vi "Disk On.vi"(0 "Notifier Name":string, 11 "Error In":errorcluster) -> (4 "Notifier Name Dup":string, 8 "Disk On?":bool, 15 "Error Out":errorcluster)   [LabVIEW 2020]
uses:
  Spinning Disk Type Defs/SD Notifer Data.ctl
  Spinning Disk Type Defs/SD Actions.ctl
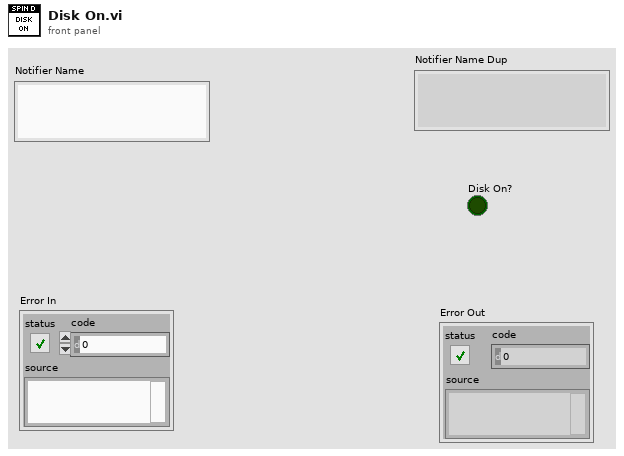
[diagram p1: front panel]
types:
  T1 = typedef "SD Notifer Data.ctl" = cluster{"Actions":T2, "Disk On?":bool, "Dichroic Pos.":i32, "Filter Wheel Pos.":i32, "Disk Pos.":i32, "Recived":bool, "Num Pos":i32[]}
  T2 = typedef "SD Actions.ctl" = enum16{"Status", "Get All Pos.", "Get Num. Pos.", "Home All", "Set Filter Wheel Pos.", "Set Disk Pos.", "Set Dichroic Pos.", "Disk On", "Disk Off", "Quit"}
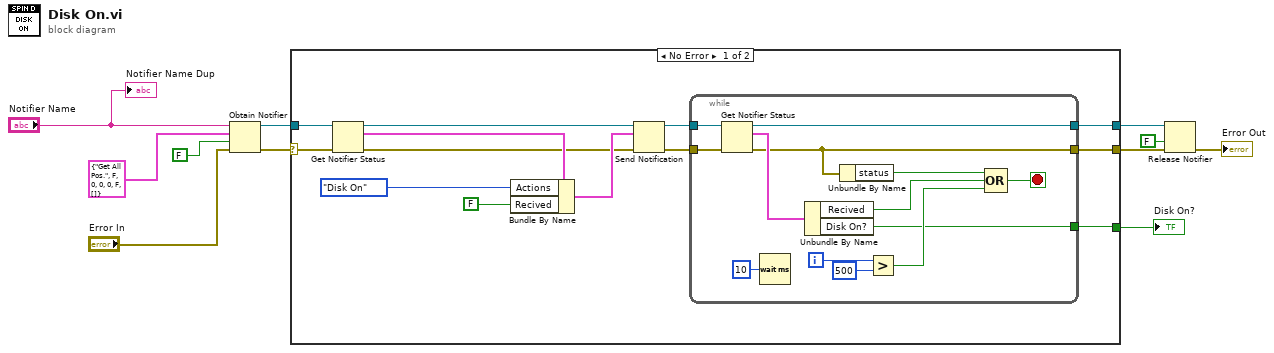
[diagram p0: block diagram]
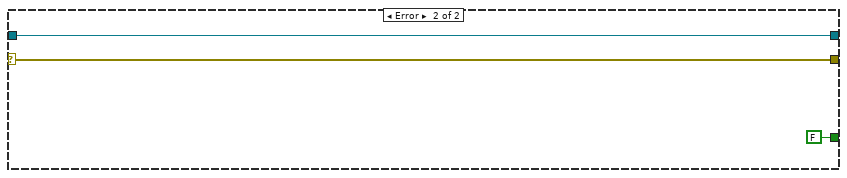
[diagram p2: hidden frame]
diagram:
  n1 = Obtain Notifier(name (unnamed)="Notifier Name", notification data type=T1 {"Actions"=enum."Get All Pos.", "Disk On?"=FALSE, "Dichroic Pos."=0, "Filter Wheel Pos."=0, "Disk Pos."=0, "Recived"=FALSE, "Num Pos"=[]} ("XLight Notifier Data"), create if not found? (T)=FALSE, error in (no error)="Error In") -> (notifier out=w7:refnum<notifier>, error out=w4:errorcluster)  [unwired: 1 out]
  n2 = case shown="No Error" w4 {
    selector: w4 -> [w23 w39]
    tunnel: w7 -> [w24 w40]
    tunnel: [w13 w40] -> w6
    tunnel: [w14 w39] -> w3
    tunnel: [w12 FALSE ("Disk On?")] -> w1
    frame No Error {
      n3 = Get Notifier Status(notifier=w24, error in (no error)=w23) -> (notifier out=w19:refnum<notifier>, current notification=w22:T1, error out=w17:errorcluster)  [unwired: 2 out]
      n4 = Bundle By Name(cluster=w22, "Actions"=SD_Actions."Disk On", "Recived"=FALSE) -> (w18:T1)
      n5 = Send Notification(notification=w18, notifier=w19, error in (no error)=w17) -> (notifier out=w16:refnum<notifier>, error out=w15:errorcluster)
      n6 = while {
        tunnel: w16 -> [w35]
        tunnel: w15 -> [w34]
        tunnel: [w28] -> w14
        tunnel: [w27] -> w13
        tunnel: [w26] -> w12
        i -> [w37]
        stop <- w29 stop-if-true
        n7 = Get Notifier Status(notifier=w35, error in (no error)=w34) -> (notifier out=w27:refnum<notifier>, current notification=w33:T1, error out=w28:errorcluster)  [unwired: 2 out]
        n8 = Wait (ms)(milliseconds to wait=u32 10) -> ()  [unwired: 1 out]
        n9 = Unbundle By Name(w33) -> ("Recived"=w32:bool, "Disk On?"=w26:bool)
        n10 = Unbundle By Name(w28) -> ("status"=w31:bool)
        n11 = Greater?(x=w37, y=500) -> (0:w30:bool)
        n12 = Compound Arithmetic op=OR(w31, w32, w30) -> (w29:bool)
      }
    }
    frame Error {
    }
  }
  "Disk On?" <- w1
  n13 = Release Notifier(notifier=w6, force destroy? (F)=FALSE, error in (no error)=w3) -> (error out=→"Error Out":errorcluster)  [unwired: 2 out]
  "Notifier Name Dup" <- "Notifier Name"
